vi "Facade.vi"(0 "Data In":T15={"Type"=enum."Tone", "Tone"={"Frequency (kHz)"=0.0, "Last Freq"=0.0, "Last Phase"=0.0}, "Pulse Train"={"Pulse width (us)"=0.0, "Pulse rate (Hz)"=0.0, "Gap (ms)"=0.0, "Polarity"=enum."POS", "PT State"={"Template"=[], "Nperiod"=0, "Index"=0, "Pulse Rate (Hz)"=0.0, "Phase (cycles)"=0.0, "Noff"=0}, "Asynch"=FALSE}, "Noise"={"InvFilt"=FALSE, "Noise"=[], "CurPt"=0, "Aweight"=FALSE, "Seed"=0, "afile"=path ""}, "File"={"Filename"=path "", "Signal"=[], "Channel"=0, "stream"=FALSE, "offset"=0, "nreps"=0, "loops"=0, "Randomize"=FALSE, "order"=[], "Seed"=0, "Tokens"=0}, "FMSweep"={"Rate (oct/s)"=0.0, "Fmin (Hz)"=0.0, "Fmax (Hz)"=0.0, "Ramp (ms)"=0.0, "Linear"=FALSE}, "Chirp Train"={"Params"={"Fmin (kHz)"=4.0, "Fmax (kHz)"=64.0, "Compensate"=FALSE, "Duration (ms)"=2.0}, "Data"={"WF"=[]}}, "Complex Tone"={"Params"={"F0 (Hz)"=0.0, "Band"={"Flow (Hz)"=0.0, "Fhigh (Hz)"=0.0}, "Phase"=enum."Cosine", "Min F0 (Hz)"=0.0, "Max F0 (Hz)"=0.0, "ContinRandPhase"=FALSE, "Max peak factor"=inf, "Max mod depth"=2.0, "MinHarmNum"=0, "MaxHarmNum"=0, "Level Mode"=enum."per component", "% jitter"=0.0}, "Data"={"Ncomp"=0, "MinHarm"=0, "Phase"=[], "Amplitude"=[], "Npts/frame"=0, "Last F0"=0.0, "Fmin"=0.0, "Fmax"=0.0, "Lslope"=0.0, "randphase"=FALSE, "overall rms"=FALSE, "fmult"=[], "jittered"=FALSE}}, "Moving Ripple"={"Params"={"Fmin"=0.0, "Fmax"=0.0, "Density"=0.0, "Velocity"=0.0, "Depth"=0.0, "Phase"=0.0, "Comp/oct"=0}, "Data"={"Freq"=[], "A"=[], "phase"=[], "Phase"=0.0}}}, 2 "Display State In":T13, 3 "Container State":T14) -> (6 "Data Out":T15={"Type"=enum."Tone", "Tone"={"Frequency (kHz)"=0.0, "Last Freq"=0.0, "Last Phase"=0.0}, "Pulse Train"={"Pulse width (us)"=0.0, "Pulse rate (Hz)"=0.0, "Gap (ms)"=0.0, "Polarity"=enum."POS", "PT State"={"Template"=[], "Nperiod"=0, "Index"=0, "Pulse Rate (Hz)"=0.0, "Phase (cycles)"=0.0, "Noff"=0}, "Asynch"=FALSE}, "Noise"={"InvFilt"=FALSE, "Noise"=[], "CurPt"=0, "Aweight"=FALSE, "Seed"=0, "afile"=path ""}, "File"={"Filename"=path "", "Signal"=[], "Channel"=0, "stream"=FALSE, "offset"=0, "nreps"=0, "loops"=0, "Randomize"=FALSE, "order"=[], "Seed"=0, "Tokens"=0}, "FMSweep"={"Rate (oct/s)"=0.0, "Fmin (Hz)"=0.0, "Fmax (Hz)"=0.0, "Ramp (ms)"=0.0, "Linear"=FALSE}, "Chirp Train"={"Params"={"Fmin (kHz)"=4.0, "Fmax (kHz)"=64.0, "Compensate"=FALSE, "Duration (ms)"=2.0}, "Data"={"WF"=[]}}, "Complex Tone"={"Params"={"F0 (Hz)"=0.0, "Band"={"Flow (Hz)"=0.0, "Fhigh (Hz)"=0.0}, "Phase"=enum."Cosine", "Min F0 (Hz)"=0.0, "Max F0 (Hz)"=0.0, "ContinRandPhase"=FALSE, "Max peak factor"=inf, "Max mod depth"=2.0, "MinHarmNum"=0, "MaxHarmNum"=0, "Level Mode"=enum."per component", "% jitter"=0.0}, "Data"={"Ncomp"=0, "MinHarm"=0, "Phase"=[], "Amplitude"=[], "Npts/frame"=0, "Last F0"=0.0, "Fmin"=0.0, "Fmax"=0.0, "Lslope"=0.0, "randphase"=FALSE, "overall rms"=FALSE, "fmult"=[], "jittered"=FALSE}}, "Moving Ripple"={"Params"={"Fmin"=0.0, "Fmax"=0.0, "Density"=0.0, "Velocity"=0.0, "Depth"=0.0, "Phase"=0.0, "Comp/oct"=0}, "Data"={"Freq"=[], "A"=[], "phase"=[], "Phase"=0.0}}}, 7 "Display State Out":T13, 8 "Action":T12)   [LabVIEW 2020, in "Waveform XCtl.xctl"]
uses:
  Waveform XCtl.xctl
  Waveform Data.ctl
  Waveform Enum.ctl
  Waveform VIs/Tone VIs/Tone Params.ctl
  Waveform VIs/Pulse Train VIs/Pulse Train Params.ctl
  Waveform VIs/Pulse Train VIs/Pulse Polarity.ctl
  Waveform VIs/Pulse Train VIs/PT-Continuous State.ctl
  Waveform VIs/Noise VIs/Noise Params.ctl
  Waveform VIs/File VIs/StimFile-Params.ctl
  Waveform VIs/FM Sweep VIs/FM Sweep Params.ctl
  Waveform VIs/Chirp Train VIs/Chirp Train.ctl
  Waveform VIs/Chirp Train VIs/Chirp Train Params.ctl
  Waveform VIs/Complex Tone VIs/CT-Params.ctl
  Waveform VIs/Complex Tone VIs/CT-Phase Enum.ctl
  Waveform VIs/Complex Tone VIs/CT-Runtime Data.ctl
  Waveform VIs/Moving Ripple VIs/Moving Ripple.ctl
  Waveform VIs/Moving Ripple VIs/Moving Ripple.Params.ctl
  Waveform VIs/Moving Ripple VIs/Moving Ripple.Data.ctl
  <vilib>/_xctls/Container State.ctl
  State.ctl
  <vilib>/_xctls/Action.ctl
  <vilib>/_xctls/XControlSupport.lvlib
panel:
  in  "Waveform":T1=enum."Tone"
  in  "Tab Control":T2(tab)
  in  "Tone Params":T3
  in  "Noise":T4
  in  "Inverse filter":bool caption="Acoustic system compensation"
  in  "A-weight":bool caption="Mouse audiogram compensation"
  in  "Pulse Train Params":T5
  in  "File Params":T8
  in  "FMSweep":T9
  in  "Chirp Train Params":T10={"Fmin (kHz)"=4.0, "Fmax (kHz)"=64.0, "Compensate"=FALSE, "Duration (ms)"=2.0}
  in  "Ripple":T11
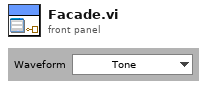
[diagram p1: front panel]
types:
  T1 = typedef "Waveform Enum.ctl" = enum16{"OFF", "Tone", "Noise", "Pulse Train", "File", "FM Sweep", "Chirp Train", "Complex Tone", "FM Tone", "Moving Ripple"}
  T2 = enum32{"OFF", "Tone", "Noise", "Pulse train", "File", "FM Sweep", "Chirp", "Ripple"}
  T3 = typedef "Tone Params.ctl" = cluster{"Frequency (kHz)":dbl, "Last Freq":dbl, "Last Phase":dbl}
  T4 = typedef "Noise Params.ctl" = cluster{"InvFilt":bool, "Noise":dbl[], "CurPt":i32, "Aweight":bool, "Seed":i32, "afile":path}
  T5 = typedef "Pulse Train Params.ctl" = cluster{"Pulse width (us)":dbl, "Pulse rate (Hz)":dbl, "Gap (ms)":dbl, "Polarity":T6, "PT State":T7, "Asynch":bool}
  T6 = typedef "Pulse Polarity.ctl" = enum16{"POS", "NEG", "POS-NEG", "NEG-POS"}
  T7 = typedef "PT-Continuous State.ctl" = cluster{"Template":dbl[], "Nperiod":i32, "Index":i32, "Pulse Rate (Hz)":dbl, "Phase (cycles)":dbl, "Noff":i32}
  T8 = typedef "StimFile-Params.ctl" = cluster{"Filename":path, "Signal":dbl[], "Channel":i32, "stream":bool, "offset":i32, "nreps":i32, "loops":i32, "Randomize":bool, "order":i32[], "Seed":i32, "Tokens":i32}
  T9 = cluster{"Rate (oct/s)":dbl, "Fmin (Hz)":dbl, "Fmax (Hz)":dbl, "Ramp (ms)":dbl, "Linear":bool}
  T10 = cluster{"Fmin (kHz)":dbl, "Fmax (kHz)":dbl, "Compensate":bool, "Duration (ms)":dbl}
  T11 = cluster{"Fmin (Hz)":dbl, "Fmax (Hz)":dbl, "Density (cyc/oct)":dbl, "Velocity (Hz)":dbl, "Depth (0-1)":dbl, "Phase (cyc)":dbl, "Comp/oct":i32}
  T12 = typedef "XControlSupport.lvlib/Action.ctl" = cluster{"Data Changed?":bool, "State Changed?":bool, "Action Name":string}
  T13 = typedef "Waveform XCtl.xctl/State.ctl" = cluster{"Numeric":dbl}
  T14 = typedef "XControlSupport.lvlib/Container State.ctl" = cluster{"Indicator?":bool, "Run Mode?":bool, " Refnum":refnum<vi>}
  T15 = typedef "Waveform XCtl.xctl/Waveform Data.ctl" = cluster{"Type":T1, "Tone":T3, "Pulse Train":T5, "Noise":T4, "File":T8, "FMSweep":T16, "Chirp Train":T17, "Complex Tone":cluster{"Params":T19, "Data":T21}, "Moving Ripple":T22}
  T16 = typedef "FM Sweep Params.ctl" = cluster{"Rate (oct/s)":dbl, "Fmin (Hz)":dbl, "Fmax (Hz)":dbl, "Ramp (ms)":dbl, "Linear":bool}
  T17 = typedef "Chirp Train.ctl" = cluster{"Params":T18, "Data":cluster{"WF":dbl[]}}
  T18 = typedef "Chirp Train Params.ctl" = cluster{"Fmin (kHz)":dbl, "Fmax (kHz)":dbl, "Compensate":bool, "Duration (ms)":dbl}
  T19 = typedef "CT-Params.ctl" = cluster{"F0 (Hz)":dbl, "Band":cluster{"Flow (Hz)":dbl, "Fhigh (Hz)":dbl}, "Phase":T20, "Min F0 (Hz)":dbl, "Max F0 (Hz)":dbl, "ContinRandPhase":bool, "Max peak factor":dbl, "Max mod depth":dbl, "MinHarmNum":i32, "MaxHarmNum":i32, "Level Mode":enum16{"per component", "overall rms"}, "% jitter":dbl}
  T20 = typedef "CT-Phase Enum.ctl" = enum16{"Cosine", "Random", "Alternating"}
  T21 = typedef "CT-Runtime Data.ctl" = cluster{"Ncomp":i32, "MinHarm":i32, "Phase":dbl[], "Amplitude":dbl[], "Npts/frame":i32, "Last F0":dbl, "Fmin":dbl, "Fmax":dbl, "Lslope":dbl, "randphase":bool, "overall rms":bool, "fmult":dbl[], "jittered":bool}
  T22 = typedef "Moving Ripple.ctl" = cluster{"Params":T23, "Data":T24}
  T23 = typedef "Moving Ripple.Params.ctl" = cluster{"Fmin":dbl, "Fmax":dbl, "Density":dbl, "Velocity":dbl, "Depth":dbl, "Phase":dbl, "Comp/oct":i32}
  T24 = typedef "Moving Ripple.Data.ctl" = cluster{"Freq":dbl[], "A":dbl[], "phase":dbl[], "Phase":dbl}
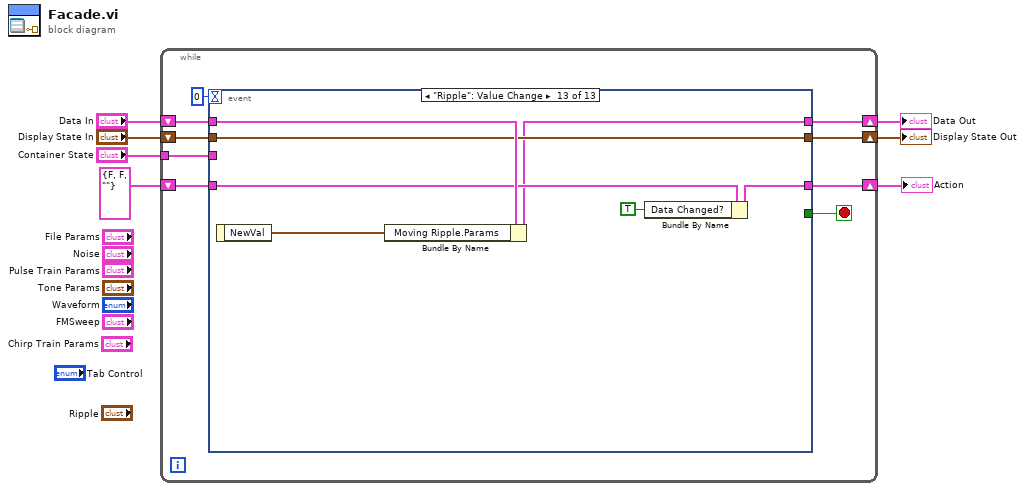
[diagram p0: block diagram]
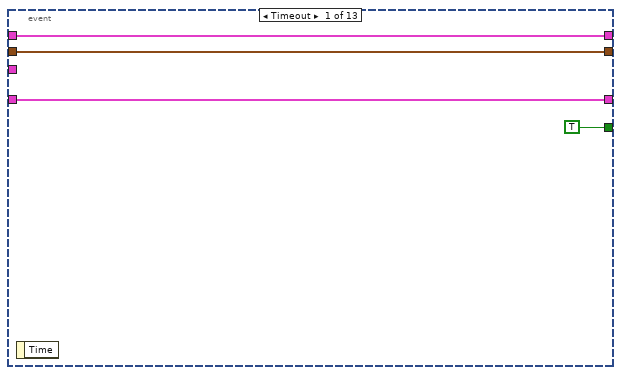
[diagram p2: hidden frame]
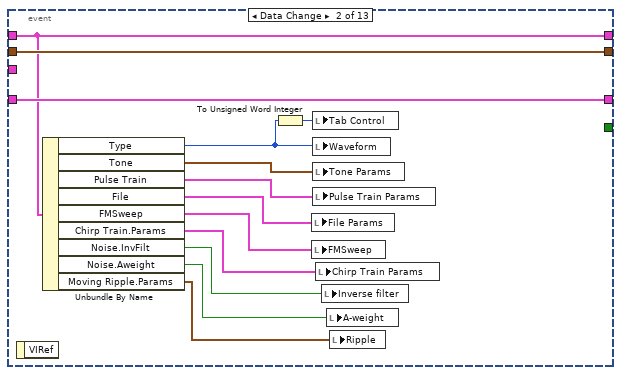
[diagram p3: hidden frame]
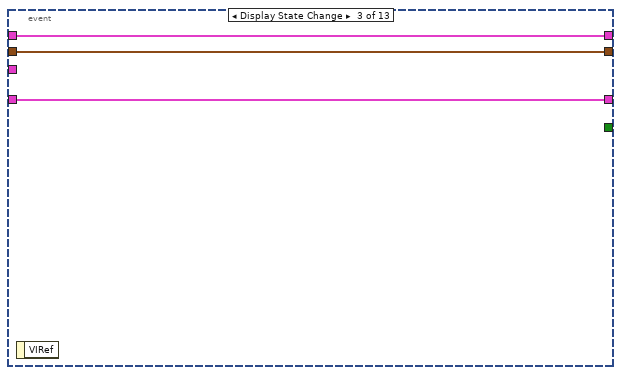
[diagram p4: hidden frame]
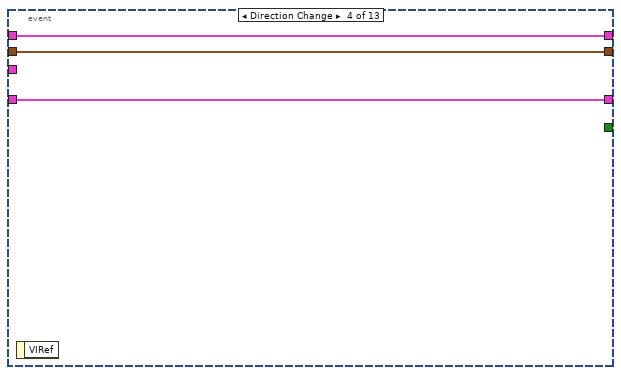
[diagram p5: hidden frame]
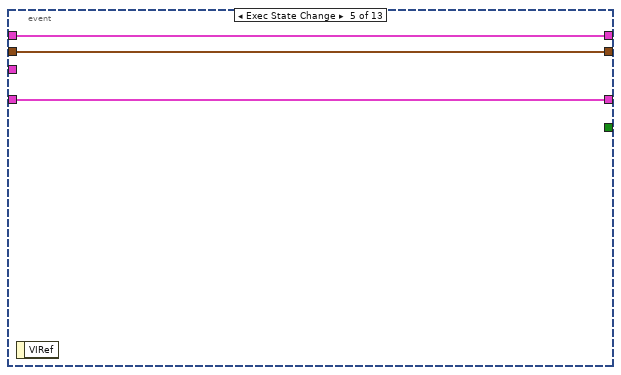
[diagram p6: hidden frame]
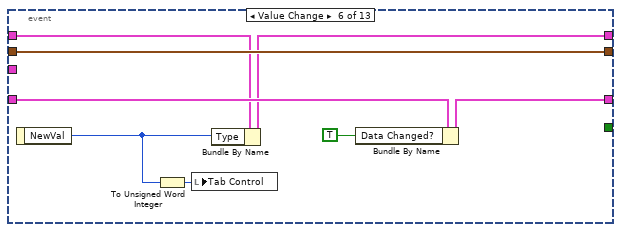
[diagram p7: hidden frame]
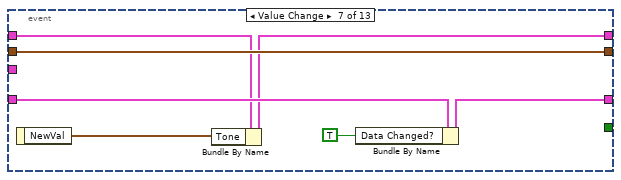
[diagram p8: hidden frame]
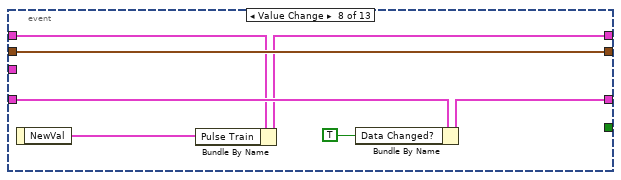
[diagram p9: hidden frame]
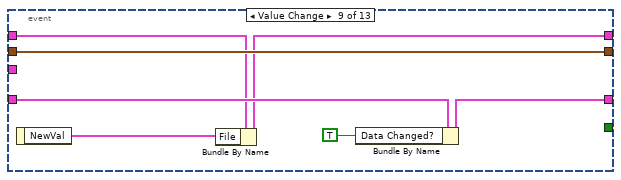
[diagram p10: hidden frame]
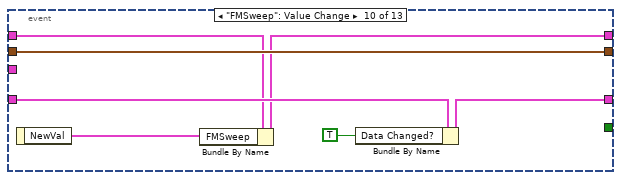
[diagram p11: hidden frame]
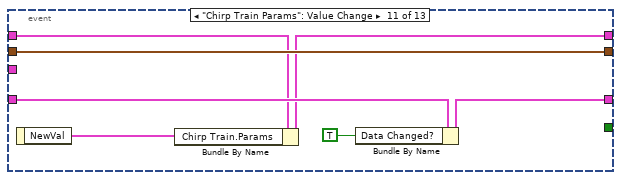
[diagram p12: hidden frame]
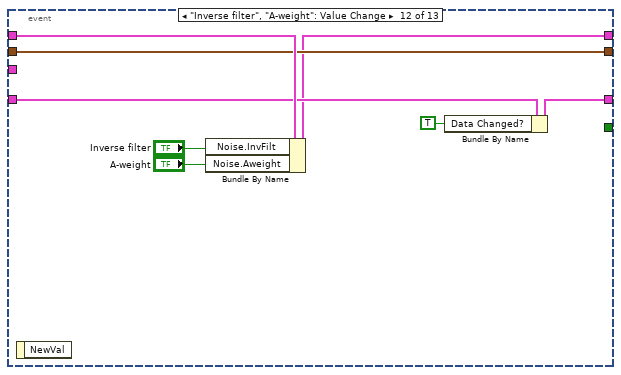
[diagram p13: hidden frame]
diagram:
  n1 = while {
    shift-right: [w15] -> w4
    shift-left: "Display State In" -> [w16]
    tunnel: "Container State" -> [w12]
    shift-right: [w10] -> w7
    shift-left: "Data In" -> [w11]
    shift-right: [w8] -> w2
    shift-left: T12 {"Data Changed?"=FALSE, "State Changed?"=FALSE, "Action Name"=""} ("Action") -> [w9]
    stop <- w14 stop-if-true
    n2 = event shown="[12] \"Ripple\": Value Change" {
      selector: _ -> [_ _ _ _ _ _ _ _ _ _ _ _ _]
      dyn-events: _ -> [_ _ _ _ _ _ _ _ _ _ _ _ _]
      timeout: 0 -> [_ _ _ _ _ _ _ _ _ _ _ _ _]
      tunnel: w16 -> [w18 w33 w36 w39 w42 w50 w57 w64 w71 w78 w85 w92 w99]
      tunnel: [w18 w33 w36 w39 w42 w50 w57 w64 w71 w78 w85 w92 w99] -> w15
      tunnel: [TRUE _ _ _ _ _ _ _ _ _ _ _ _] -> w14
      tunnel: w12 -> [_ _ _ _ _ _ _ _ _ _ _ _ _]
      tunnel: w11 -> [w17 w31 w35 w38 w41 w46 w53 w60 w67 w74 w81 w93 w100]
      tunnel: [w17 w31 w35 w38 w41 w45 w52 w59 w66 w73 w80 w88 w95] -> w10
      tunnel: [w19 w32 w34 w37 w40 w47 w54 w61 w68 w75 w82 w90 w97] -> w8
      tunnel: w9 -> [w19 w32 w34 w37 w40 w49 w56 w63 w70 w77 w84 w91 w98]
      event Timeout {
        n3 = event-data() -> ()  [unwired: 1 in, 1 out]
      }
      event Data Change {
        n4 = event-data() -> ()  [unwired: 1 in, 1 out]
        n5 = Unbundle By Name(w31) -> ("Type"=w27:T1, "Tone"=w30:T3, "Pulse Train"=w29:T5, "File"=w26:T8, "FMSweep"=w25:T16, "Chirp Train.Params"=w24:T18, "Noise.InvFilt"=w23:bool, "Noise.Aweight"=w22:bool, "Moving Ripple.Params"=w21:T23)
        n6 = To Unsigned Word Integer(number=w27) -> (unsigned 16bit integer=w28:u16)
        n7 = local write "File Params"(w26) -> ()
        n8 = local write "FMSweep"(w25) -> ()
        n9 = local write "Tab Control"(w28) -> ()
        n10 = local write "Waveform"(w27) -> ()
        n11 = local write "Tone Params"(w30) -> ()
        n12 = local write "Pulse Train Params"(w29) -> ()
        n13 = local write "Chirp Train Params"(w24) -> ()
        n14 = local write "Inverse filter"(w23) -> ()
        n15 = local write "A-weight"(w22) -> ()
        n16 = local write "Ripple"(w21) -> ()
      }
      event Display State Change {
        n17 = event-data() -> ()  [unwired: 1 in, 1 out]
      }
      event Direction Change {
        n18 = event-data() -> ()  [unwired: 1 in, 1 out]
      }
      event Exec State Change {
        n19 = event-data() -> ()  [unwired: 1 in, 1 out]
      }
      event Value Change {
        n20 = event-data() -> ("NewVal"=w43:T1)  [unwired: 1 in]
        n21 = To Unsigned Word Integer(number=w43) -> (unsigned 16bit integer=w44:u16)
        n22 = local write "Tab Control"(w44) -> ()
        n23 = Bundle By Name(cluster=w46, "Type"=w43) -> (w45:T15)
        n24 = Bundle By Name(cluster=w49, "Data Changed?"=TRUE) -> (w47:T12)
      }
      event Value Change {
        n25 = event-data() -> ("NewVal"=w51:T3)  [unwired: 1 in]
        n26 = Bundle By Name(cluster=w53, "Tone"=w51) -> (w52:T15)
        n27 = Bundle By Name(cluster=w56, "Data Changed?"=TRUE) -> (w54:T12)
      }
      event Value Change {
        n28 = event-data() -> ("NewVal"=w58:T5)  [unwired: 1 in]
        n29 = Bundle By Name(cluster=w60, "Pulse Train"=w58) -> (w59:T15)
        n30 = Bundle By Name(cluster=w63, "Data Changed?"=TRUE) -> (w61:T12)
      }
      event Value Change {
        n31 = event-data() -> ("NewVal"=w65:T8)  [unwired: 1 in]
        n32 = Bundle By Name(cluster=w67, "File"=w65) -> (w66:T15)
        n33 = Bundle By Name(cluster=w70, "Data Changed?"=TRUE) -> (w68:T12)
      }
      event "FMSweep": Value Change {
        n34 = event-data() -> ("NewVal"=w72:T9)  [unwired: 1 in]
        n35 = Bundle By Name(cluster=w74, "FMSweep"=w72) -> (w73:T15)
        n36 = Bundle By Name(cluster=w77, "Data Changed?"=TRUE) -> (w75:T12)
      }
      event "Chirp Train Params": Value Change {
        n37 = event-data() -> ("NewVal"=w79:T10)  [unwired: 1 in]
        n38 = Bundle By Name(cluster=w81, "Chirp Train.Params"=w79) -> (w80:T15)
        n39 = Bundle By Name(cluster=w84, "Data Changed?"=TRUE) -> (w82:T12)
      }
      event "Inverse filter", "A-weight": Value Change {
        n40 = event-data() -> ()  [unwired: 1 in, 1 out]
        n41 = Bundle By Name(cluster=w93, "Noise.InvFilt"="Inverse filter", "Noise.Aweight"="A-weight") -> (w88:T15)
        n42 = Bundle By Name(cluster=w91, "Data Changed?"=TRUE) -> (w90:T12)
      }
      event "Ripple": Value Change {
        n43 = event-data() -> ("NewVal"=w94:T11)  [unwired: 1 in]
        n44 = Bundle By Name(cluster=w100, "Moving Ripple.Params"=w94) -> (w95:T15)
        n45 = Bundle By Name(cluster=w98, "Data Changed?"=TRUE) -> (w97:T12)
      }
    }
  }
  "Display State Out" <- w4
  "Data Out" <- w7
  "Action" <- w2
